vi "Get Index.vi"(11 "File Path Control":path) -> (3 "Index":i32)   [LabVIEW 2016]
panel:
  out "match substring":string
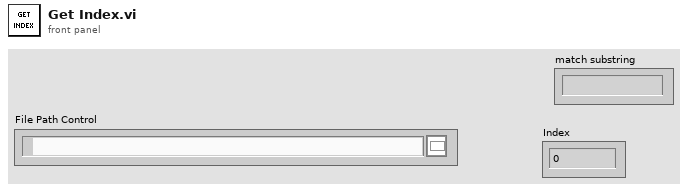
[diagram p1: front panel]
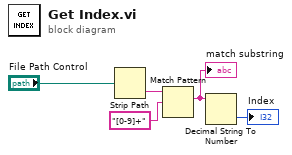
[diagram p0: block diagram]
diagram:
  n1 = Strip Path(path="File Path Control") -> (name=w4:string)  [unwired: 1 out]
  n2 = Match Pattern(string=w4, regular expression="[0-9]+") -> (match substring=w2:string)  [unwired: 1 in, 3 out]
  "match substring" <- w2
  n3 = Decimal String To Number(string=w2) -> (number=→"Index":i32)  [unwired: 2 in, 1 out]
